vi "CryoServer Cmd Piper Passthrough.vi"(8 "error in (no error)":errorcluster, 9 "Piper Command":string, 10 "Piper Board ID (Hex)":u32 format="%x", 11 "connection ID":refnum<k5>) -> (0 "error out":errorcluster, 1 "Response":string, 2 "cmd str":string, 3 "connection ID out":refnum<k5>)   [LabVIEW 2024, in "CryoServer.lvclass"]
uses:
  CryoServer.lvclass
  <vilib>/JDP Science/JSONtext/Next JSON Value.vi
  <vilib>/JDP Science/JSONtext/String Subset.vi
  <vilib>/JDP Science/JSONtext/Parsing/Advance past next JSON Value (inlined COPY).vi
  <vilib>/JDP Science/JSONtext/Parsing/Advance past whitespace.vi
  <vilib>/JDP Science/JSONtext/Parsing/Advance past String.vi
  <vilib>/JDP Science/JSONtext/Parsing/Advance past Number.vi
  <vilib>/JDP Science/JSONtext/Parsing/Advance past Line Ending.vi
  <vilib>/JDP Science/JSONtext/Parsing/Parse Full Path or Item Name.vi
  <vilib>/JDP Science/JSONtext/Parsing/Advance past Array.vi
  <vilib>/JDP Science/JSONtext/Parsing/Advance past Object.vi
  <vilib>/JDP Science/JSONtext/support/Error Cluster From Code.vi
  <vilib>/JDP Science/JSONtext/Offset/Find Item Locations by Path.vi
  <vilib>/JDP Science/JSONtext/JSONtext.lvlib
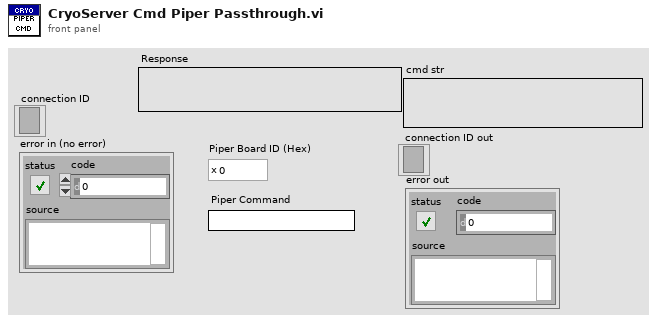
[diagram p1: front panel]
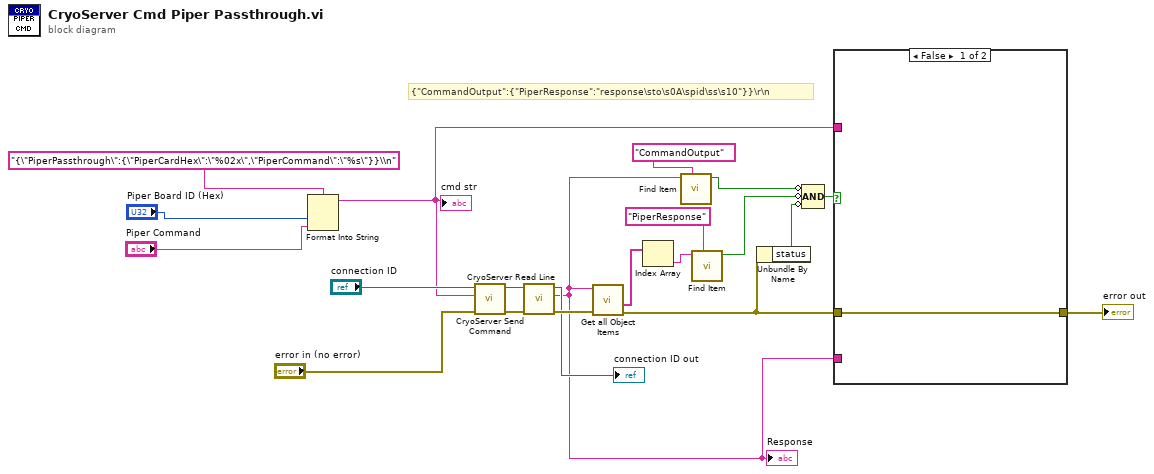
[diagram p0: block diagram]
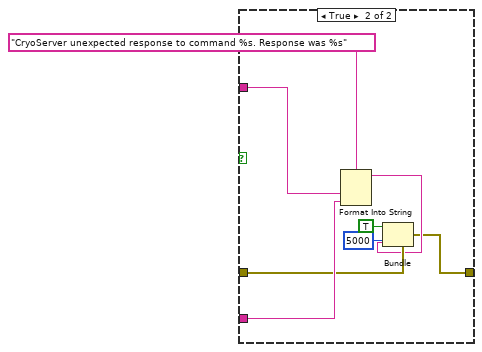
[diagram p2: hidden frame]
diagram:
  # "{\"CommandOutput\":{\"PiperResponse\":\"response\\sto\\s0A\\spid\\ss\\s10\"}}\\r\\n"
  n1 = Format Into String(format string="{\"PiperPassthrough\":{\"PiperCardHex\":\"%02x\",\"PiperCommand\":\"%s\"}}\\n", "Piper Board ID (Hex)", "Piper Command") -> (resulting string=w4:string)  [unwired: 2 in, 1 out]
  "cmd str" <- w4
  n2 = call "CryoServer Send Command.vi"("error in (no error)"="error in (no error)", "command string"=w4, "connection ID"="connection ID") -> ("error out"=w16:errorcluster, "connection ID out"=w15:refnum<k5>)  [unwired: 6 in, 1 out]
  n3 = call "CryoServer Read Line.vi"("error in (no error)"=w16, "connection ID"=w15) -> ("error out"=w8:errorcluster, "data out"=w3:string, "connection ID out"=→"connection ID out":refnum<k5>)  [unwired: 7 in]
  "Response" <- w3
  n4 = call <vilib>:"Get all Object Items.vi"("error in (no error)"=w8, "JSON"=w3) -> ("error out"=w2:errorcluster, "<JSON>"=w13:string[])  [unwired: 6 in, 2 out]
  n5 = Index Array(array=w13) -> (element=w12:string)  [unwired: 1 in]
  n6 = call <vilib>:"Find Item.vi"("$Path or Item Name"="CommandOutput" ("y"), "JSON"=w3) -> ("Found"=w10:bool)  [unwired: 6 in, 3 out]
  n7 = call <vilib>:"Find Item.vi"("$Path or Item Name"="PiperResponse", "JSON"=w12) -> ("Found"=w9:bool)  [unwired: 6 in, 3 out]
  n8 = Unbundle By Name(w2) -> ("status"=w7:bool)
  n9 = Compound Arithmetic op=AND(invert w10, invert w9, invert w7) -> (w6:bool)
  n10 = case shown="False" w6 {
    tunnel: w4 -> [_ w29]
    tunnel: w3 -> [_ w28]
    tunnel: w2 -> [w22 w27]
    tunnel: [w22 w23] -> w1
    frame False {
    }
    frame True {
      n11 = Format Into String(format string="CryoServer unexpected response to command %s. Response was %s", w29, w28) -> (resulting string=w24:string)  [unwired: 2 in, 1 out]
      n12 = Bundle(cluster=w27, "status"=TRUE, "code"=5000, "source"=w24) -> (w23:errorcluster)
    }
  }
  "error out" <- w1
